vi "Create Step Update Map.vi"(11 "Settings UI in":refnum<class "Settings UI.lvclass">) -> (2 "Step Update Map out":T1(c390), 3 "Settings UI out":refnum<class "Settings UI.lvclass">)   [LabVIEW 2020, in "Output Sequencer.lvlib" / "Settings UI.lvclass"]
uses:
  Settings UI.lvclass
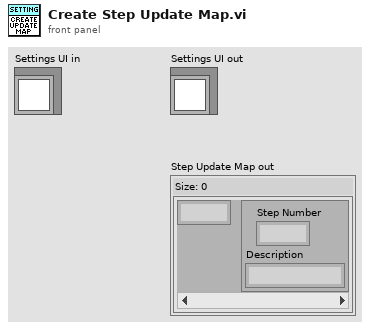
[diagram p1: front panel]
types:
  T1 = map{i32, cluster{"Step Number":i32, "Description":string}}
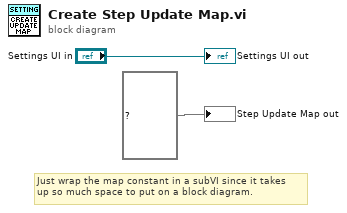
[diagram p0: block diagram]
diagram:
  # "Just wrap the map constant in a subVI since it takes\nup so much space to put on a block diagram."
  "Settings UI out" <- "Settings UI in"
  "Step Update Map out" <- T1 {} ("map")
